vi "lib macpath_to_unixstring.vi"(4 "Path":path) -> (1 "Output String":string)   [LabVIEW 2016]
doc: "This Changes Mac file separaters to /"
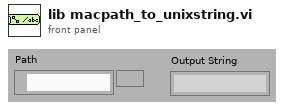
[diagram p1: front panel]
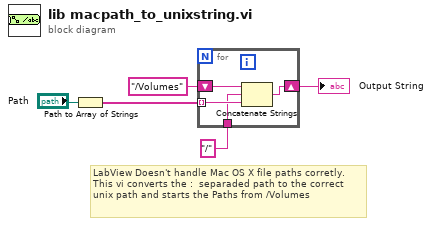
[diagram p0: block diagram]
diagram:
  # "LabView Doesn't handle Mac OS X file paths corretly. This vi converts the :  separaded path to the correct unix path and starts the Paths from /Volumes"
  n1 = Path to Array of Strings(0:"Path") -> (2:w1:string[])  [unwired: 1 out]
  n2 = for {
    tunnel: w1 -> [w7] mode=indexing
    shift-right: [w9] -> w4
    shift-left: "/Volumes" -> [w8]
    tunnel: "/" -> [w6]
    n3 = Concatenate Strings(w8, w6, w7) -> (w9:string)
  }
  "Output String" <- w4
